vi "set ID.vi"(10 "ID":string, 11 "task in":refnum<class "task.lvclass">) -> (3 "task out":refnum<class "task.lvclass">)   [LabVIEW 2013, in "task.lvclass"]
uses:
  task.lvclass
  task.lvclass/task.ctl
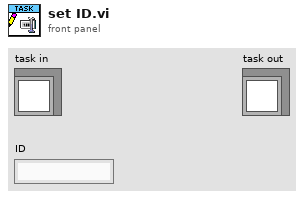
[diagram p1: front panel]
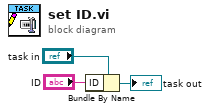
[diagram p0: block diagram]
diagram:
  n1 = Bundle By Name(cluster="task in", "ID"="ID") -> (→"task out":refnum<class "task.lvclass">)
